vi "test_date.vi"() -> ()   [LabVIEW 2017]
panel:
  out "current time":timestamp
  out "concatenated string":string
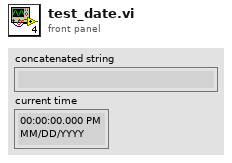
[diagram p1: front panel]
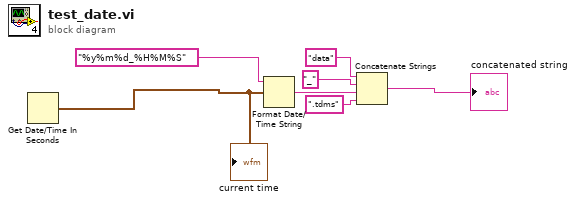
[diagram p0: block diagram]
diagram:
  n1 = Get Date/Time In Seconds() -> (seconds since 1Jan1904=w1:timestamp)
  "current time" <- w1
  n2 = Format Date/Time String(time format string (%c)="%y%m%d_%H%M%S", seconds (now)=w1) -> (date/time string=w6:string)  [unwired: 1 out]
  n3 = Concatenate Strings("data" ("string"), "_" ("string"), w6, ".tdms" ("string")) -> (→"concatenated string":string)
